vi "global_stop.vi"() -> ()   [LabVIEW 2019]
panel:
  in  "정지 버튼":bool=TRUE
  # "눌러놓고 시작!!"
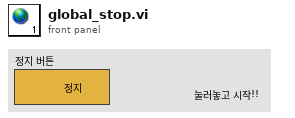
[diagram p1: front panel]
diagram:
